vi "Window Direct Message.vi"(8 "error in (no error)":errorcluster, 10 "Message Cluster":T1, 11 "Server in":refnum<class "Server.lvclass">) -> (0 "error out":errorcluster, 3 "Server out":refnum<class "Server.lvclass">)   [LabVIEW 2020, in "Server.lvlib" / "Server.lvclass"]
uses:
  Server.lvclass
  Application Control/Message.ctl
  Server.lvclass/Server.ctl
  Chat Room Model/Chat Room Model Messages/ReceiveNewMessage Msg/ReceiveNewMessage Msg.lvclass
  3eb30432-9714-485c-8ebb-9ec49c9eae9e.vi
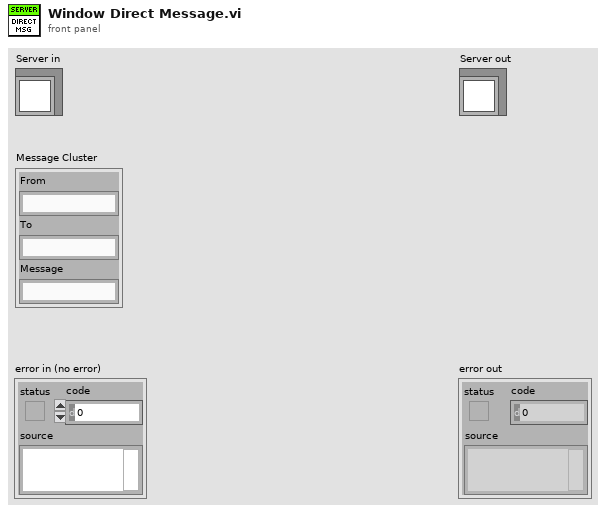
[diagram p1: front panel]
types:
  T1 = typedef "Message.ctl" = cluster{"From":string, "To":string, "Message":string}
  T2 = typedef "Chat Room Model.lvlib/Chat Room Model.lvclass/User Info.ctl" = cluster{"Name":string, "Status":string}
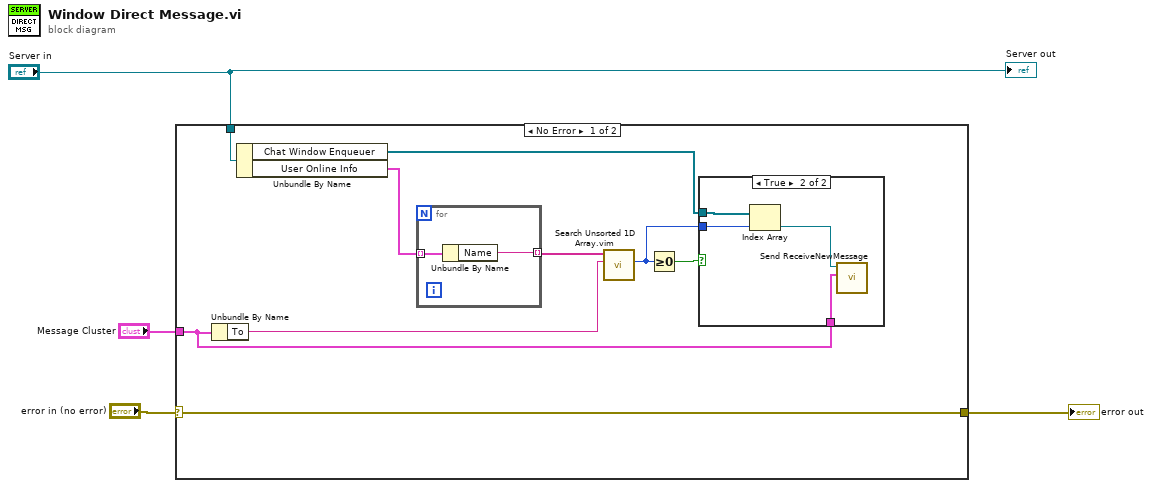
[diagram p0: block diagram]
diagram:
  n1 = case shown="No Error" "error in (no error)" {
    selector: "error in (no error)" -> [w5 w20]
    tunnel: "Message Cluster" -> [w6 _]
    tunnel: "Server in" -> [w13 _]
    tunnel: [w5 w20] -> w1
    frame No Error {
      n2 = Unbundle By Name(w6) -> ("To"=w10:string)
      n3 = Unbundle By Name(w13) -> ("Chat Window Enqueuer"=w8:refnum<class "Message Enqueuer.lvclass">[], "User Online Info"=w12:T2[])
      n4 = for {
        tunnel: w12 -> [w19] mode=indexing
        tunnel: [w18] -> w11 mode=indexing
        n5 = Unbundle By Name(w19) -> ("Name"=w18:string)
      }
      n6 = call "Search Unsorted 1D Array.vim"("element"=w10, "unsorted 1D array"=w11) -> ("index of element"=w7:i32)  [unwired: 9 in]
      n7 = Greater Or Equal To 0?(x=w7) -> (x >= 0?=w9:bool)
      n8 = case shown="True" w9 {
        tunnel: w8 -> [_ w17]
        tunnel: w7 -> [_ w16]
        tunnel: w6 -> [_ w15]
        frame False {
        }
        frame True {
          n9 = Index Array(array=w17, index=w16) -> (element=w14:refnum<class "Message Enqueuer.lvclass">)
          n10 = call "Send ReceiveNewMessage.vi"("Message Cluster"=w15, "Message Enqueuer"=w14) -> ()  [unwired: 8 in, 2 out]
        }
      }
    }
    frame Error {
    }
  }
  "error out" <- w1
  "Server out" <- "Server in"
